vi "shift_points.vi"() -> (0 "Torque/MPH":cluster{dbl[], dbl[]}[](graph), 1 "Intercepts":dbl[](array[numeric]))   [LabVIEW 2025]
panel:
  out "RPM/MPH":cluster{dbl[], "all rows":dbl[]}[](graph)
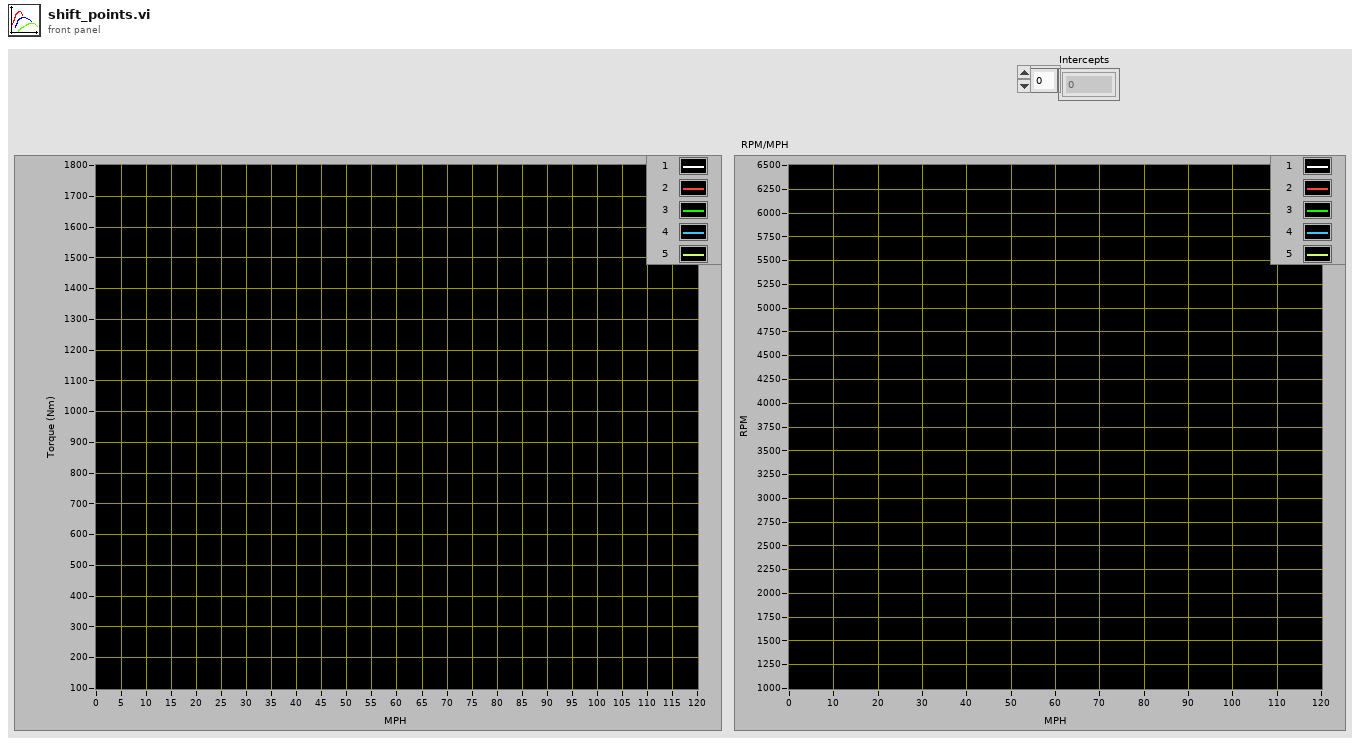
[diagram p1: front panel]
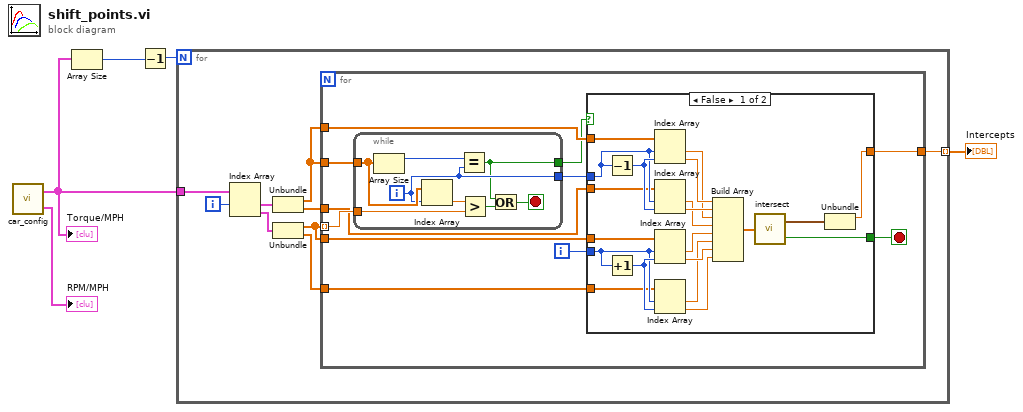
[diagram p0: block diagram]
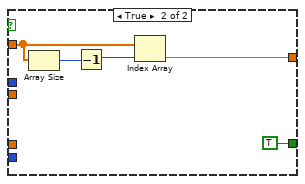
[diagram p2: hidden frame]
diagram:
  n1 = call "car_config.vi"() -> ("Torque/MPH"=w3:cluster{dbl[], dbl[]}[], "RPM/MPH"=→"RPM/MPH":cluster{dbl[], "all rows":dbl[]}[])  [unwired: 1 in]
  "Torque/MPH" <- w3
  n2 = Array Size(array=w3) -> (size(s)=w4:i32)
  n3 = Decrement(x=w4) -> (x-1=w5:i32)
  n4 = for {
    N: w5 -> [_]
    tunnel: w3 -> [w7]
    tunnel: [w9] -> w1 mode=indexing
    i -> [w6]
    n5 = Index Array(array=w7, index #1=w6) -> (element #1=w14:cluster{dbl[], dbl[]}, element #2=w8:cluster{dbl[], dbl[]})  [unwired: 1 in]
    n6 = Unbundle(w14) -> (w13:dbl[], w11:dbl[])
    n7 = Unbundle(w8) -> (w12:dbl[], w10:dbl[])
    n8 = for {
      tunnel: w13 -> [w24]
      tunnel: w12 -> [w25] mode=indexing
      tunnel: w13 -> [w16]
      tunnel: w11 -> [w18]
      tunnel: w12 -> [w20]
      tunnel: w10 -> [w22]
      tunnel: [w23] -> w9
      i -> [w21]
      stop <- w17 stop-if-true
      n9 = while {
        tunnel: w25 -> [w58]
        tunnel: w24 -> [w56]
        tunnel: [w53] -> w19
        tunnel: [w51] -> w15
        i -> [w53]
        stop <- w55 stop-if-true
        n10 = Array Size(array=w56) -> (size(s)=w54:i32)
        n11 = Index Array(array=w56, index=w53) -> (element=w57:dbl)
        n12 = Equal?(x=w54, y=w53) -> (x = y?=w51:bool)
        n13 = Greater?(x=w57, y=w58) -> (0:w52:bool)
        n14 = Or(x=w51, y=w52) -> (x .or. y?=w55:bool)
      }
      n15 = case shown="False" w15 {
        tunnel: [w27 w46] -> w23
        tunnel: w22 -> [w28 _]
        tunnel: w21 -> [w29 _]
        tunnel: w20 -> [w30 _]
        tunnel: w19 -> [w32 _]
        tunnel: w18 -> [w31 _]
        tunnel: [w26 TRUE ("valid")] -> w17
        tunnel: w16 -> [w33 w48]
        frame False {
          n16 = Decrement(x=w32) -> (x-1=w45:i32)
          n17 = Increment(x=w29) -> (x+1=w44:i32)
          n18 = Index Array(array=w33, index #1=w32, index #2=w45) -> (element #1=w41:dbl, element #2=w43:dbl)
          n19 = Index Array(array=w31, index #1=w32, index #2=w45) -> (element #1=w40:dbl, element #2=w42:dbl)
          n20 = Index Array(array=w30, index #1=w29, index #2=w44) -> (element #1=w39:dbl, element #2=w38:dbl)
          n21 = Index Array(array=w28, index #1=w29, index #2=w44) -> (element #1=w37:dbl, element #2=w36:dbl)
          n22 = Build Array(w43, w42, w41, w40, w39, w37, w38, w36) -> (w35:dbl[])
          n23 = call "intersect.vi"("coords"=w35) -> ("intersect"=w34:cluster{"x*y":dbl, "x*y":dbl}, "valid"=w26:bool)
          n24 = Unbundle(w34) -> ("x*y"=w27:dbl)  [unwired: 1 out]
        }
        frame True {
          n25 = Array Size(array=w48) -> (size(s)=w50:i32)
          n26 = Decrement(x=w50) -> (x-1=w49:i32)
          n27 = Index Array(array=w48, index=w49) -> (element=w46:dbl)
        }
      }
    }
  }
  "Intercepts" <- w1
